vi "Add Correction Table Entries.vi"(8 "error in (no error)":errorcluster, 9 "Entries":cluster{"Frequency":dbl, "Attenuation":dbl}[](array[cluster]) {"Attenuation" format="%#_6f"; "Frequency" format="%#_6e"}, 10 "Correction Table (\"Table1\")":string="Table1", 11 "VISA resource name":refnum<visa-resource-name>) -> (0 "error out":errorcluster, 3 "VISA resource name out":refnum<visa-resource-name>)   [LabVIEW 2020, in "Rohde&Schwarz CMXP Base.lvlib"]
doc: "Adds entries to an existing correction table. Specify at least one parameter pair of Frequency and Attenuation.\n\nAttribute:\n-\n\nRemote-control command:\nADD:SYSTem:ATTenuation:CTABle"
uses:
  <instrlib>/Rohde&Schwarz CMXP Base/Rohde&Schwarz CMXP Base.lvlib
  <instrlib>/Rohde&Schwarz CMXP Base/Private/rsidr_core.llb/rsidr_core.lvlib
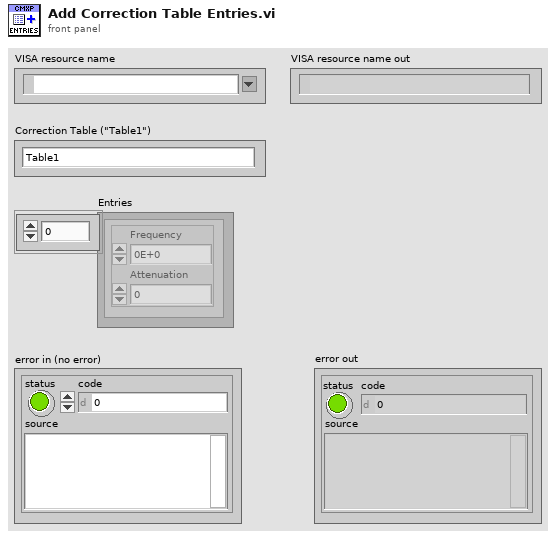
[diagram p1: front panel]
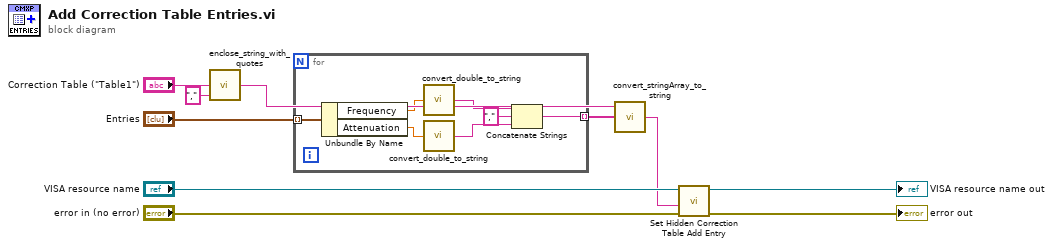
[diagram p0: block diagram]
diagram:
  n1 = call <instrlib>:"enclose_string_with_quotes.vi"("String after"=",", "String to enclose"="Correction Table (\"Table1\")") -> ("String out"=w3:string)  [unwired: 3 in]
  n2 = for {
    tunnel: "Entries" -> [w17] mode=indexing
    tunnel: [w11] -> w4 mode=indexing
    n3 = Unbundle By Name(w17) -> ("Frequency"=w15:dbl, "Attenuation"=w16:dbl)
    n4 = call <instrlib>:"convert_double_to_string.vi"("double in"=w15) -> ("string out"=w13:string)  [unwired: 4 in]
    n5 = call <instrlib>:"convert_double_to_string.vi"("double in"=w16) -> ("string out"=w12:string)  [unwired: 4 in]
    n6 = Concatenate Strings(w13, "," ("string"), w12) -> (w11:string)
  }
  n7 = call <instrlib>:"convert_stringArray_to_string.vi"("string array in"=w4, "String to add before (\"\")"=w3) -> ("string out"=w2:string)  [unwired: 3 in]
  n8 = call "Set Hidden Correction Table Add Entry"("error in (no error)"="error in (no error)", "Hidden Correction Table Add Entry ()"=w2, "instrument handle"="VISA resource name") -> ("error out"=→"error out":errorcluster, "instrument handle out"=→"VISA resource name out":refnum<visa-resource-name>)  [unwired: 7 in]
